vi "Compile Protocol.vi"(8 "error in (no error)":errorcluster, 11 "Python Protocol in":refnum<class "Python Protocol.lvclass">) -> (0 "error out":errorcluster, 3 "Python Protocol out":refnum<class "Python Protocol.lvclass">)   [LabVIEW 2013, in "Python Protocol.lvlib" / "Python Protocol.lvclass"]
uses:
  Python Protocol.lvclass
  <userlib>/_OpenG.lib/labpython/labpython.llb/PYTHON Set Float Data__ogtk.vi
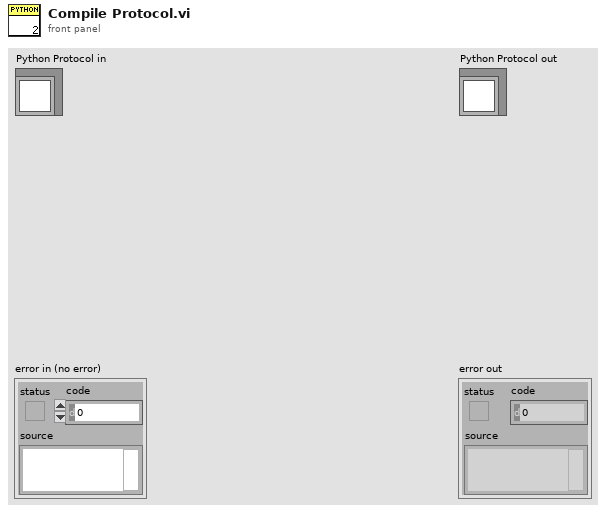
[diagram p1: front panel]
types:
  T1 = typedef "PYTHON Session Refnum__ogtk.ctl" = refnum<k1>
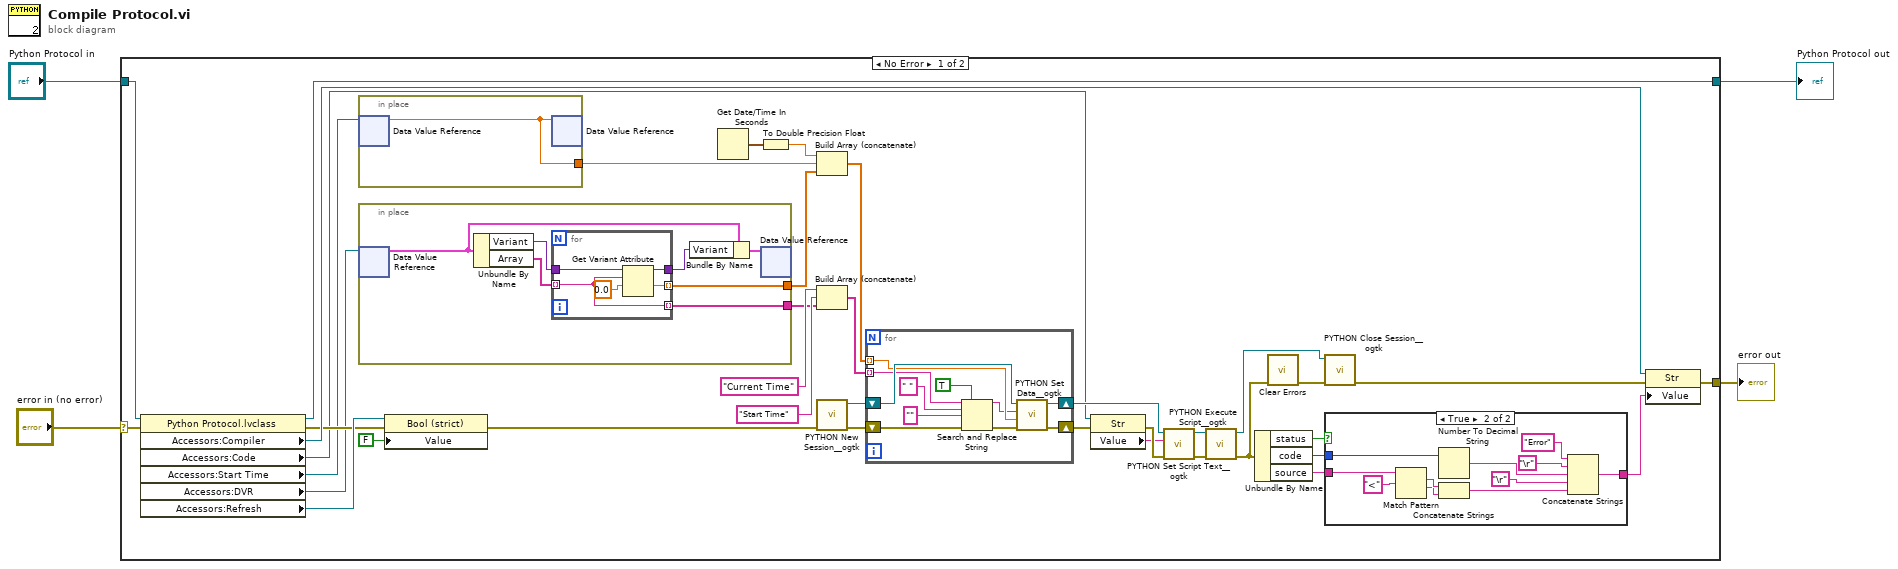
[diagram p0: block diagram]
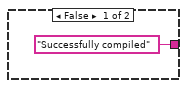
[diagram p2: hidden frame]
diagram:
  n1 = case shown="No Error" "error in (no error)" {
    selector: "error in (no error)" -> [w27 w79]
    tunnel: [w26 w79] -> w3
    tunnel: [w31 w78] -> w1
    tunnel: "Python Protocol in" -> [w32 w78]
    frame No Error {
      n2 = property class="Python Protocol.lvclass"(reference=w32, error in=w27) -> (reference out=w31:refnum<class "Python Protocol.lvclass">, error out=w28:errorcluster, "Accessors:Compiler"=w30:refnum<vi>, "Accessors:Code"=w6:refnum<vi>, "Accessors:Start Time"=w10:refnum<data-value>, "Accessors:DVR"=w9:refnum<data-value>, "Accessors:Refresh"=w29:refnum<vi>)
      n3 = in-place {
        in-place-border: [w42] -> w14
        n4 = in-place-dvr #1(w10) -> (w42:dbl)  [unwired: 1 out]
        n5 = in-place-dvr #1(w42) -> ()  [unwired: 2 out]
      }
      n6 = in-place {
        in-place-border: [w44] -> w12
        in-place-border: [w43] -> w11
        n7 = in-place-dvr #2(w9) -> (w47:cluster{"Array":string[], "Variant":variant})  [unwired: 1 out]
        n8 = Unbundle By Name(w47) -> ("Variant"=w49:variant, "Array"=w48:string[])
        n9 = for {
          tunnel: w49 -> [w54]
          tunnel: w48 -> [w50] mode=indexing
          tunnel: [w52] -> w45
          tunnel: [w51] -> w44 mode=indexing
          tunnel: [w50] -> w43 mode=indexing
          n10 = Get Variant Attribute(Variant=w54, name=w50, default value (empty Variant)=0.0) -> (duplicate Variant=w52:variant, value=w51:dbl)  [unwired: 1 in, 2 out]
        }
        n11 = Bundle By Name(cluster=w47, "Variant"=w45) -> (w46:cluster{"Array":string[], "Variant":variant})
        n12 = in-place-dvr #2(w46) -> ()  [unwired: 2 out]
      }
      n13 = property class="Bool (strict)"(reference=w29, error in=w28, "Value"=FALSE) -> (error out=w5:errorcluster)  [unwired: 1 out]
      n14 = Get Date/Time In Seconds() -> (seconds since 1Jan1904=w22:timestamp)
      n15 = To Double Precision Float(number=w22) -> (double precision float=w13:dbl)
      n16 = Build Array (concatenate)(w13, w14, w12) -> (w17:dbl[])
      n17 = Build Array (concatenate)("Current Time", "Start Time" ("element"), w11) -> (w21:string[])
      n18 = call <userlib>:"PYTHON New Session__ogtk.vi"("error in (no error)"=w5) -> ("error out"=w25:errorcluster, "Python Session"=w24:T1)  [unwired: 5 in]
      n19 = for {
        tunnel: w21 -> [w55] mode=indexing
        shift-right: [w64] -> w20
        shift-left: w24 -> [w63]
        shift-right: [w65] -> w23
        shift-left: w25 -> [w62]
        tunnel: w17 -> [w57] mode=indexing
        n20 = Search and Replace String(replace all?=TRUE ("replace all? (F)"), input string=w55, search string=" ", replace string="" ("replace string (\"\")"), error in=w62) -> (result string=w56:string, error out=w61:errorcluster)  [unwired: 3 in, 2 out]
        n21 = call-poly <userlib>:"PYTHON Set Data__ogtk.vi"("error in (no error)"=w61, "value"=w57, "variable name"=w56, "Python Session in"=w63) -> ("error out"=w65:errorcluster, "Python Session out"=w64:T1)  [unwired: 2 in]
      }
      n22 = property class="Str"(reference=w6, error in=w23) -> (error out=w19:errorcluster, "Value"=w18:string)  [unwired: 1 out]
      n23 = call <userlib>:"PYTHON Set Script Text__ogtk.vi"("error in (no error)"=w19, "script text"=w18, "Python Session in"=w20) -> ("error out"=w8:errorcluster, "Python Session out"=w7:T1)  [unwired: 3 in]
      n24 = call <userlib>:"PYTHON Execute Script__ogtk.vi"("error in (no error)"=w8, "Python Session in"=w7) -> ("error out"=w34:errorcluster, "Python Session out"=w36:T1)  [unwired: 4 in]
      n25 = Unbundle By Name(w34) -> ("status"=w39:bool, "code"=w41:i32, "source"=w40:string)
      n26 = call <vilib>:"Clear Errors.vi"("error in (no error)"=w34) -> ("error out"=w37:errorcluster)  [unwired: 6 in]
      n27 = call <userlib>:"PYTHON Close Session__ogtk.vi"("error in (no error)"=w37, "Python Session in"=w36) -> ("error out"=w35:errorcluster)  [unwired: 5 in]
      n28 = case shown="True" w39 {
        tunnel: w41 -> [_ w77]
        tunnel: w40 -> [_ w71]
        tunnel: ["Successfully compiled" w74] -> w38
        frame False {
        }
        frame True {
          n29 = Match Pattern(string=w71, regular expression="<") -> (match substring=w69:string, after substring=w68:string)  [unwired: 1 in, 2 out]
          n30 = Number To Decimal String(number=w77) -> (decimal integer string=w76:string)  [unwired: 1 in]
          n31 = Concatenate Strings(w69, w68) -> (w67:string)
          n32 = Concatenate Strings("Error" ("string"), "\r", w76, "\r", w67) -> (w74:string)
        }
      }
      n33 = property class="Str"(reference=w30, error in=w35, "Value"=w38) -> (error out=w26:errorcluster)  [unwired: 1 out]
    }
    frame Error {
    }
  }
  "error out" <- w3
  "Python Protocol out" <- w1
